vi "Read From RDMA Buffer.vi"(8 "error in":errorcluster, 9 "timeout ms (25000)":i32=25000 format="%d ms", 10 "rdma session":refnum<k21>, 11 "RDMA Transceiver in":refnum<class "RDMA Transceiver.lvclass">) -> (0 "error out":errorcluster, 1 "timed out?":bool, 2 "data":string, 3 "RDMA Transceiver out":refnum<class "RDMA Transceiver.lvclass">)   [LabVIEW 2020, in "RDMA.lvlib" / "RDMA Transceiver.lvclass"]
doc: "Reads data from RDMA buffer."
uses:
  RDMA Transceiver.lvclass
  RDMA Transceiver.lvclass/RDMA Transceiver.ctl
  <vilib>/rdma/rdma.llb/RDMA Acquire Received Buffer U8.vi
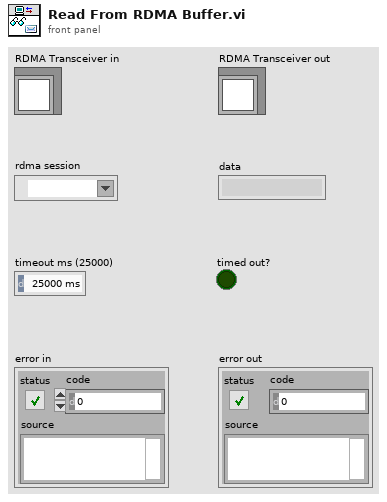
[diagram p1: front panel]
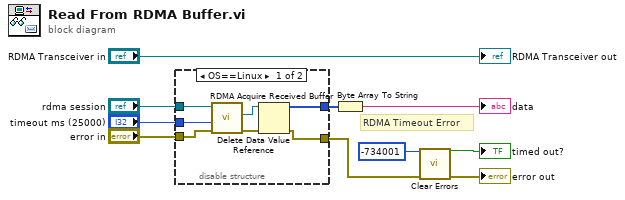
[diagram p0: block diagram]
diagram:
  # "RDMA Timeout Error"
  n1 = disable-structure shown="OS==Linux" {
    disable-tunnel: "timeout ms (25000)" -> [w17 _]
    disable-tunnel: [w15 _] -> w5
    disable-tunnel: [w14 _] -> w1
    disable-tunnel: "rdma session" -> [w11 _]
    disable-tunnel: "error in" -> [w13 _]
    frame condition #0 (active) {
      n2 = call-poly <vilib>:"RDMA Acquire Received Buffer.vi"("error in"=w13, "timeout (ms)"=w17, "rdma session in"=w11) -> ("error out"=w12:errorcluster, "edvr"=w16:refnum<data-value>)  [unwired: 6 in, 1 out]
      n3 = Delete Data Value Reference(data value reference=w16, error in=w12) -> (data value=w14:u8[], error out=w15:errorcluster)
    }
    frame condition #1 {
    }
  }
  n4 = Byte Array To String(unsigned byte array=w1) -> (string=→"data":string)
  n5 = call <vilib>:"Clear Errors.vi"("error in (no error)"=w5, "specific error code to clear (0: all)"=-734001) -> ("error out"=→"error out":errorcluster, "specific error cleared?"=→"timed out?":bool)  [unwired: 4 in]
  "RDMA Transceiver out" <- "RDMA Transceiver in"
